vi "GMS_a_Decimal.vi"(1 "Segundos":i32, 2 "Minutos":i32, 3 "Grados":i32) -> (0 "Decimal":dbl)   [LabVIEW 2020]
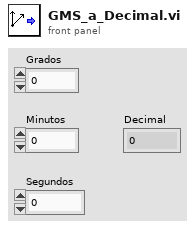
[diagram p1: front panel]
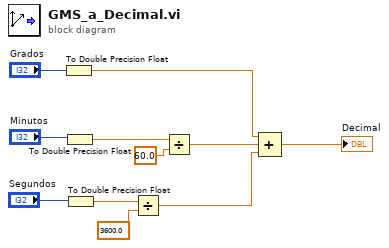
[diagram p0: block diagram]
diagram:
  n1 = To Double Precision Float(number="Grados") -> (double precision float=w5:dbl)
  n2 = To Double Precision Float(number="Minutos") -> (double precision float=w8:dbl)
  n3 = To Double Precision Float(number="Segundos") -> (double precision float=w6:dbl)
  n4 = Divide(x=w6, y=3600.0) -> (x/y=w3:dbl)
  n5 = Divide(x=w8, y=60.0) -> (x/y=w4:dbl)
  n6 = Compound Arithmetic op=ADD(w5, w4, w3) -> (→"Decimal":dbl)
